vi "Stop Autostop Nested Actors.vi"(8 "error in (no error)":errorcluster, 11 "Actor in":refnum<class "Actor.lvclass">) -> (0 "error out":errorcluster, 3 "Actor out":refnum<class "Actor.lvclass">)   [LabVIEW 2020, in "Actor Framework.lvlib" / "Actor.lvclass"]
doc: "<p>(<strong>Filename</strong>: <span class=\"dnl\">Actor Framework.lvlib:Actor.lvclass:Stop Autostop Nested Actors.vi</span>)</p>\n\n<p>Sends a normal Stop message to any auto-stop nested actors that were launched by an actor but have not yet sent back their Last Ack messages. Use this VI when you want to stop all of an actor's nested actors, but not the actor itself.</p>"
uses:
  Actor.lvclass
  Actor.lvclass/Actor.ctl
  Message Enqueuer/Message Enqueuer.lvclass/Message Enqueuer.ctl
  Message Enqueuer/Enqueue.vi
  Stop Msg/Stop Msg.lvclass
  C:/justACS/Actor Framework/Core/ActorFramework/Message/Message.lvclass
  Message Priority Queue/Priority Enqueue.vi
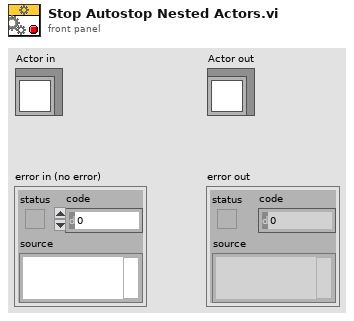
[diagram p1: front panel]
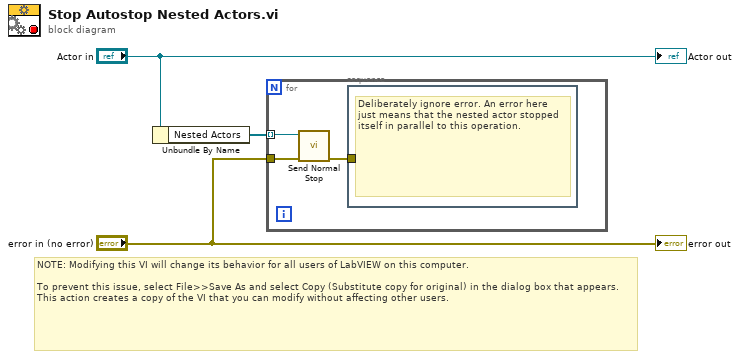
[diagram p0: block diagram]
diagram:
  # "NOTE: Modifying this VI will change its behavior for all users of LabVIEW on this computer.\n\nTo prevent this issue, select File>>Save As and select Copy (Substitute copy for original) in the dialog box that appears. This action creates a copy of the VI that you can modify without affecting other users."
  n1 = Unbundle By Name("Actor in") -> ("Nested Actors"=w3:refnum<class "Message Enqueuer.lvclass">[])
  n2 = for {
    tunnel: w3 -> [w6] mode=indexing
    tunnel: "error in (no error)" -> [w5]
    n3 = call "Send Normal Stop.vi"("error in (no error)"=w5, "Message Enqueuer"=w6) -> ("error out"=w4:errorcluster)  [unwired: 9 in]
    n4 = stacked-sequence {
      tunnel: w4 -> [_]
      frame #0 {
        # "Deliberately ignore error. An error here just means that the nested actor stopped itself in parallel to this operation."
      }
    }
  }
  "error out" <- "error in (no error)"
  "Actor out" <- "Actor in"
